vi "Write All Stderr.vi"(8 "Error In":errorcluster, 10 "Data":u8[](array[numeric]), 11 "Channel In":refnum<class "Channel.lvclass">) -> (0 "Error Out":errorcluster, 1 "Timed Out?":bool, 2 "Write Count":u64, 3 "Channel Out":refnum<class "Channel.lvclass">)   [LabVIEW 2021, in "Field_RnD_Services_LIBSSH2_Toolkit.lvlib" / "Channel.lvclass"]
doc: "Writes binary data to the STDERR stream of the SSH channel represented by this Channel object until all of the data (bytes) are written. If the binary data is larger than 30KB, then the data is written in 30KB chunks, or blocks, until the <B>Write Count</B> equals the <B>Data</B> array size."
uses:
  Channel.lvclass
  Channel.lvclass/Channel.ctl
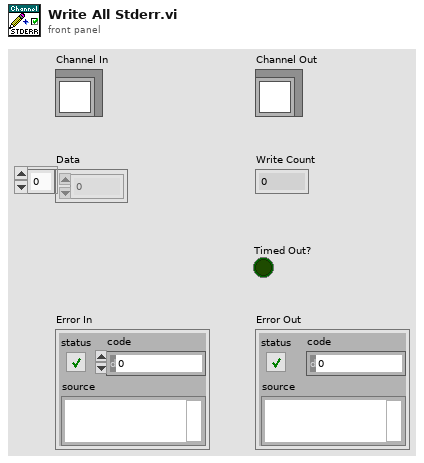
[diagram p1: front panel]
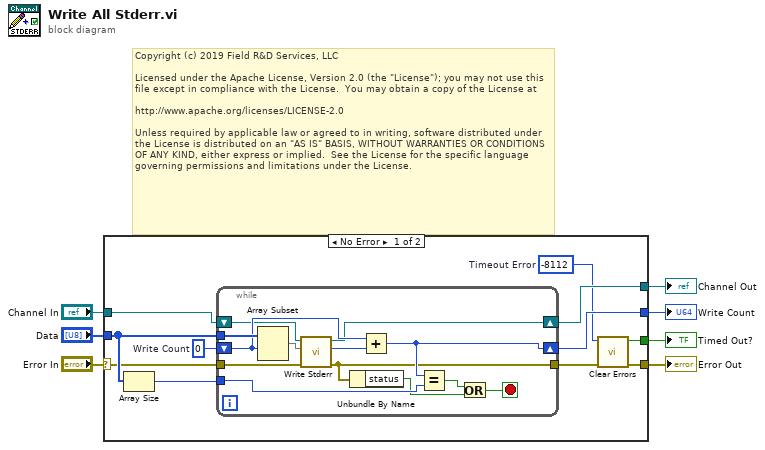
[diagram p0: block diagram]
diagram:
  # "Copyright (c) 2019 Field R&D Services, LLC\n\nLicensed under the Apache License, Version 2.0 (the \"License\"); you may not use this file except in compliance with the License.  You may obtain a copy of the License at\n\nhttp://www.apache.org/licenses/LICENSE-2.0\n\nUnless required by applicable law or agreed to in writing, software distributed under the License is distributed on an \"AS IS\" BASIS, WITHOUT WARRANTIES OR CONDITIONS OF ANY KIND, either express or implied.  See the License for the specific language governing permissions and limitations under the License."
  n1 = case shown="No Error" "Error In" {
    selector: "Error In" -> [w13 w32]
    tunnel: "Data" -> [w16 _]
    tunnel: "Channel In" -> [w15 w33]
    tunnel: [w14 w33] -> w5
    tunnel: [w10 w32] -> w4
    tunnel: [w12 _] -> w2
    tunnel: [w8 _] -> w1
    frame No Error {
      w9 = -8112  # Timeout Error
      w17 = u64 0  # Write Count
      n2 = Array Size(array=w16) -> (size(s)=w18:i32)
      n3 = while {
        tunnel: w16 -> [w31]
        shift-right: [w23] -> w14
        shift-left: w15 -> [w24]
        tunnel: w18 -> [w28]
        shift-right: [w29] -> w12
        shift-left: w17 -> [w30]
        tunnel: w13 -> [w20]
        tunnel: [w21] -> w11
        stop <- w25 stop-if-true
        n4 = Array Subset(array=w31, index=w30) -> (w19:u8[])  [unwired: 1 in]
        n5 = call "Write Stderr.vi"("Error In"=w20, "Data"=w19, "Channel In"=w24) -> ("Error Out"=w21:errorcluster, "Write Count"=w22:u64, "Channel Out"=w23:refnum<class "Channel.lvclass">)  [unwired: 6 in]
        n6 = Unbundle By Name(w21) -> ("status"=w26:bool)
        n7 = Add(x=w30, y=w22) -> (x+y=w29:u64)
        n8 = Equal?(x=w29, y=w28) -> (x = y?=w27:bool)
        n9 = Or(x=w27, y=w26) -> (x .or. y?=w25:bool)
      }
      n10 = call <vilib>:"Clear Errors.vi"("error in (no error)"=w11, "specific error code to clear (0: all)"=w9) -> ("error out"=w10:errorcluster, "specific error cleared?"=w8:bool)  [unwired: 4 in]
    }
    frame Error {
    }
  }
  "Channel Out" <- w5
  "Error Out" <- w4
  "Write Count" <- w2
  "Timed Out?" <- w1
